vi "Run RT Sequence Pass Fail Test.vi"(4 "Gateway IP Address":string, 5 "Timeout (ms)":dbl=10000.0, 6 "Target (\"\": Auto-assign)":string, 7 "Sequence File Path":path, 8 "ParamTypes":string[](array[string]), 9 "ParamValues":string[](array[string]), 10 "ParamNames":string[](array[string]), 11 "Sequence Context":refnum<k7>) -> (0 "error out":errorcluster, 2 "PassFail":bool, 3 "Report Text":string)   [LabVIEW 2013, in "RTSequenceVIs.lvlib"]
doc: "Executes a single pass of a real-time sequence giving the defined parameter names, values, and types. Outputs a pass/fail value based on the boolean return value."
uses:
  RTSequenceVIs.lvlib
  <vilib>/NI Veristand/Execution/SequenceExecutionInterface/Sequence Execution State.ctl
  NationalInstruments.VeriStand.DataTypes
  <vilib>/NI Veristand/Execution/SequenceExecutionInterface/NI_VS Sequence Execution Interface.lvlib
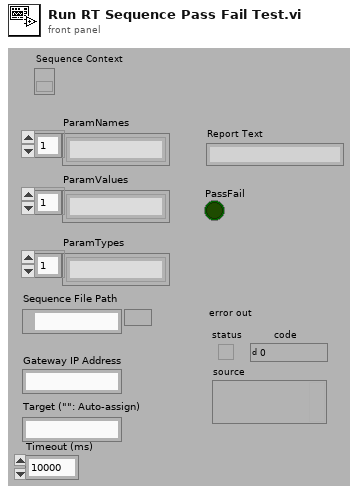
[diagram p1: front panel]
types:
  T1 = typedef "NI_VS Sequence Execution Interface.lvlib/Sequence Input Assignment Ref.ctl" = refnum<k24>
  T2 = typedef "NI_VS Sequence Execution Interface.lvlib/Sequence Call Ref.ctl" = refnum<k24>
  T3 = typedef "NI_VS Sequence Execution Interface.lvlib/Stimulus Profile Session Ref.ctl" = refnum<k24>
  T4 = typedef "TestStand - Status Monitor.ctl" = cluster{"Sequence Context":refnum<k7>, "Execution":refnum<k7>, "Termination Monitor":refnum<k7>}
  T5 = typedef "NI_VS Sequence Execution Interface.lvlib/Sequence Execution State.ctl" = enum16{"Idle", "Running", "SingleStepping", "Paused", "Stopped"}
  T6 = typedef "NI_VS Sequence Execution Interface.lvlib/Data Value Ref.ctl" = refnum<k24>
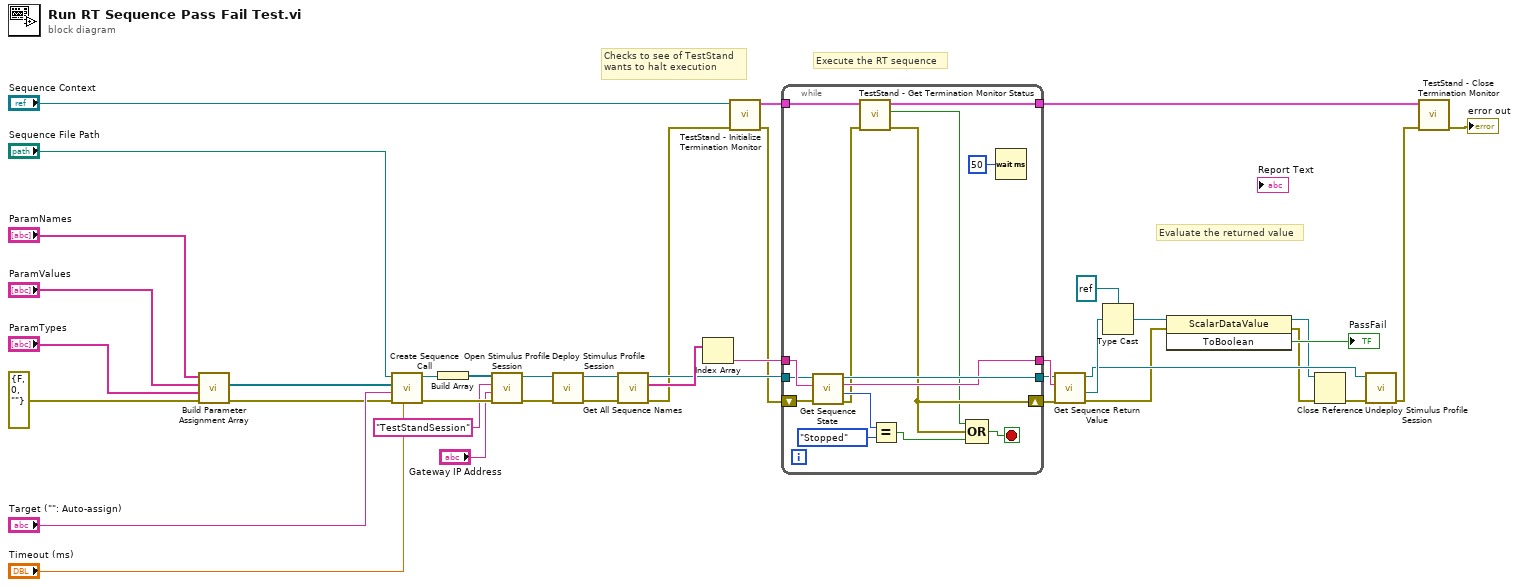
[diagram p0: block diagram]
diagram:
  # "Checks to see of TestStand\nwants to halt execution"
  # "Evaluate the returned value"
  # "Execute the RT sequence"
  n1 = call "Build Parameter Assignment Array.vi"("error in (no error)"=errorcluster {"status"=FALSE, "code"=0, "source"=""}, "ParamTypes"="ParamTypes", "ParamValues"="ParamValues", "ParamNames"="ParamNames") -> ("error out"=w6:errorcluster, "Sequence Parameter Assignment refs"=w5:T1[])  [unwired: 6 in]
  n2 = call <vilib>:"Create Sequence Call.vi"("Timeout ms (10000)"="Timeout (ms)", "error in (no error)"=w6, "Target (\"\": Auto-assign)"="Target (\"\": Auto-assign)", "Parameter Assignments"=w5, "Sequence File Path"="Sequence File Path") -> ("error out"=w40:errorcluster, "Sequence Call Ref"=w34:T2)  [unwired: 5 in]
  n3 = Build Array(w34) -> (w38:T2[])
  n4 = call <vilib>:"Open Stimulus Profile Session.vi"("error in (no error)"=w40, "Gateway IP Address (\"\": localhost)"="Gateway IP Address", "Session Name"="TestStandSession", "Sequence Calls"=w38) -> ("error out"=w36:errorcluster, "Session Ref"=w37:T3)  [unwired: 6 in]
  n5 = call <vilib>:"Deploy Stimulus Profile Session.vi"("error in (no error)"=w36, "Session Ref in"=w37) -> ("error out"=w33:errorcluster, "Session Ref out"=w32:T3)  [unwired: 7 in, 1 out]
  n6 = call <vilib>:"Get All Sequence Names.vi"("error in (no error)"=w33, "Session Ref in"=w32) -> ("error out"=w14:errorcluster, "Sequence Names out"=w31:string[], "Session Ref out"=w29:T3)  [unwired: 7 in]
  n7 = Index Array(array=w31) -> (element=w30:string)  [unwired: 1 in]
  n8 = call <vilib>:"TestStand - Initialize Termination Monitor.vi"("error in (no error)"=w14, "Sequence Context In"="Sequence Context") -> ("error out"=w13:errorcluster, "Status Monitor Out"=w12:T4)  [unwired: 8 in]
  n9 = while {
    tunnel: w30 -> [w55]
    tunnel: w29 -> [w54]
    shift-right: [w43] -> w23
    shift-left: w13 -> [w53]
    tunnel: [w48] -> w22
    tunnel: [w46] -> w28
    tunnel: w12 -> [w45]
    tunnel: [w41] -> w11
    stop <- w49 stop-if-true
    n10 = call <vilib>:"Get Sequence State.vi"("error in (no error)"=w53, "Sequence Name"=w55, "Session Ref in"=w54) -> ("error out"=w44:errorcluster, "State"=w52:T5, "Sequence Name out"=w46:string, "Session Ref out"=w48:T3)  [unwired: 5 in]
    n11 = call <vilib>:"TestStand - Get Termination Monitor Status.vi"("error in (no error)"=w44, "Status Monitor In"=w45) -> ("error out"=w43:errorcluster, "Terminating or Aborting"=w42:bool, "Status Monitor Out"=w41:T4)  [unwired: 7 in]
    n12 = Equal?(x=w52, y=Sequence_Execution_State."Stopped" ("State")) -> (x = y?=w50:bool)
    n13 = Compound Arithmetic op=OR(w42, w43, w50) -> (w49:bool)
    n14 = Wait (ms)(milliseconds to wait=u32 50 ("millisecond multiple")) -> ()  [unwired: 1 out]
  }
  n15 = call <vilib>:"Get Sequence Return Value.vi"("error in (no error)"=w23, "Sequence Name"=w28, "Session Ref in"=w22) -> ("error out"=w20:errorcluster, "Data Value Ref"=w27:T6, "Session Ref out"=w21:T3)  [unwired: 5 in, 1 out]
  n16 = Type Cast(type=refnum<k24> refnum ("Node"), x=w27) -> (*(type *) &x=w25:refnum<k24>)
  n17 = invoke class="ScalarDataValue" method="ToBoolean"(reference=w25, error in=w20) -> (reference out=w17:refnum<k24>, error out=w19:errorcluster, "ToBoolean"=→"PassFail":bool)  [unwired: 1 in]
  n18 = Close Reference(reference=w17, error in (no error)=w19) -> (error out=w18:errorcluster)
  n19 = call <vilib>:"Undeploy Stimulus Profile Session.vi"("error in (no error)"=w18, "Session Ref in"=w21) -> ("error out"=w9:errorcluster)  [unwired: 8 in, 1 out]
  n20 = call <vilib>:"TestStand - Close Termination Monitor.vi"("error in (no error)"=w9, "Status Monitor In"=w11) -> ("error out"=→"error out":errorcluster)  [unwired: 9 in]
